vi "Test Cycle.vi"() -> ()   [LabVIEW 2018, in "TLMB.lvlib"]
uses:
  Projects/TLMB.lvlib
  Common/LabVIEW GEA2 Toolkit/GEA3/type defs/Source_Destination.ctl
  Common/LabVIEW GEA2 Toolkit/GEA3/type defs/ERD Read Data In.ctl
  Common/LabVIEW GEA2 Toolkit/GEA3/type defs/Data Type.ctl
  type defs/Drive Cycle Engine Request State.ctl
  type defs/Motor Control Without Stop Start.ctl
  Common/LabVIEW GEA2 Toolkit/GEA3/type defs/ERD Write Data In.ctl
  C:/Users/iallatyp/Desktop/New folder/GEA3/library/GEA2_Toolkit.lvlib
panel:
  in  "Spray Rinse Time (s)":dbl=120.0 caption="Delay Time (s)"
  in  "Intermediate Spin Time":dbl=120.0 caption="Delay Time (s)"
  in  "Agitate Time (s)":dbl=30.0 caption="Delay Time (s)"
  in  "Final Spin Time (s)":dbl=180.0 format="%#_13g"
  out "Error Out":errorcluster={"status"=TRUE, "code"=1172, "source"="Invoke Node Error calling method GeaCommunication.GeaBus.Read, (System.ArgumentNullException: Key cannot be null.\r\nParameter name: key) <append><b>System.ArgumentNullException</b> in LabVIEW_GEA2_Toolkit.lvlibp:GEA2 Send and Receive Message.vi->LabVIEW_GEA2_Toolkit.lvlibp:GEA2 Write ERD.vi->Drive Cycle Engine Request State ERD.vi->Test Cycle.vi"}
  in  "Target Gallons":dbl=4.0
  in  "Error In":errorcluster
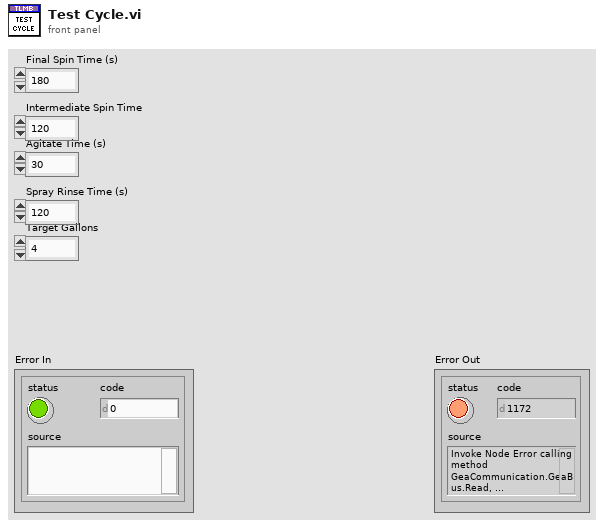
[diagram p1: front panel]
types:
  T1 = enum16{"EQ (==)", "NE (!=)", "GT (>)", "LT (<)", "GE (>=)", "LE (<=)", "GTLT(> <)", "GELE (>= <=)", "GELT (>= <)", "GTLE (> <=)", "LTGT (< >)", "LEGE (<= >=)", "LEGT (<= >)", "LTGE (< >=)", "No Comparison"}
  T2 = typedef "GEA2_Toolkit.lvlib/ERD Read Data In.ctl" = cluster{"ERD Number":u16, "Data Type":T3}
  T3 = typedef "GEA2_Toolkit.lvlib/Data Type.ctl" = enum16{"string", "boolean", "uint8_t", "uint16_t", "uint32_t", "uint64_t", "int8_t", "int16_t", "int32_t", "int64_t"}
  T4 = enum16{"ALL OFF", "Cold Valve", "Hot Valve", "Fabric Softener Valve", "Spray Rinse Valve", "Hot and Cold Valve"}
  T5 = typedef "GEA2_Toolkit.lvlib/ERD Write Data In.ctl" = cluster{"ERD Number":u16, "Data Type":T3, "Data":string}
  T6 = typedef "TLMB.lvlib/Drive Cycle Engine Request State.ctl" = enum16{"Start", "Stop", "Pause", "Resume", "Select"}
  T7 = typedef "TLMB.lvlib/Motor Control Without Stop Start.ctl" = cluster{"Speed (RPM)":i16, "Motor Profile Mode":u16, "Acceleration":i16, "Angle (Degrees)":i16, "Amplitude (%)\n-CCW +CW":i16}
  T8 = typedef "GEA2_Toolkit.lvlib/Source_Destination.ctl" = cluster{"Source":u8, "Destination":u8}
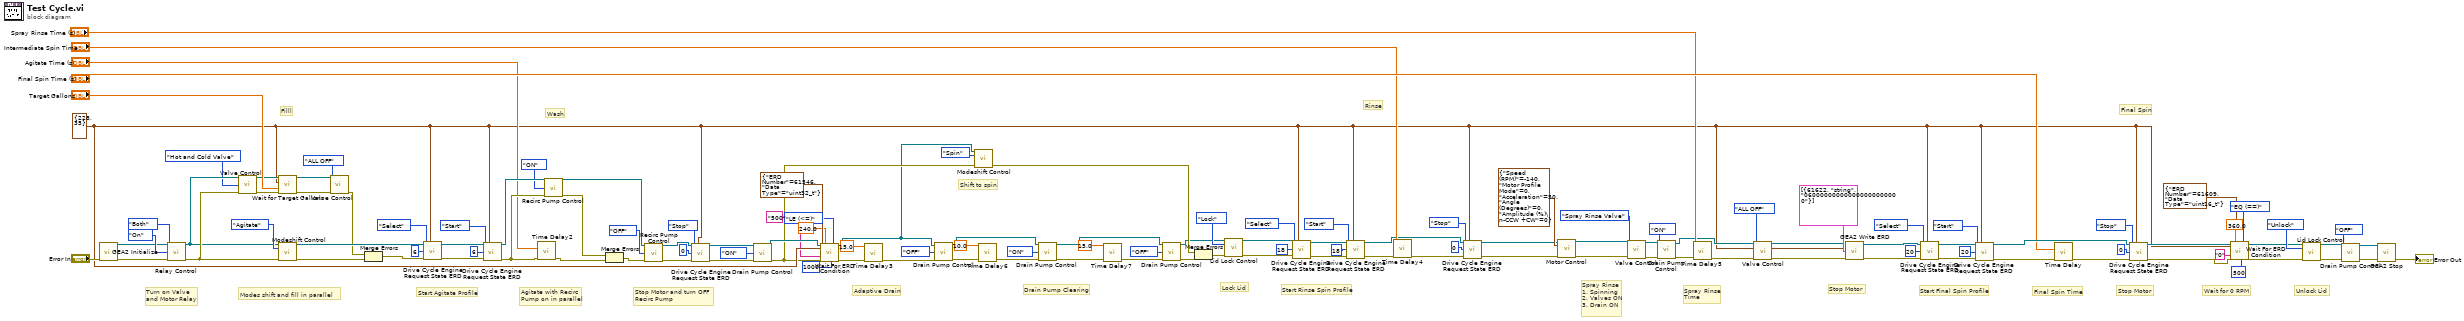
[diagram p0: block diagram]
diagram:
  w30 = T8 {"Source"=228, "Destination"=35} ("GEA Inputs")
  # "Drain Pump Clearing"
  # "Spray Rinse\n1. Spinning\n2. Valves ON\n3. Drain ON"
  # "Spray Rinse\nTime"
  # "Stop Motor"
  # "Start Rinse Spin Profile"
  # "Filll"
  # "Wash"
  # "Rinse"
  # "Final Spin"
  # "Final Spin Time"
  # "Unlock Lid"
  # "Stop Motor"
  # "Lock Lid"
  # "Shift to spin"
  # "Adaptive Drain"
  # "Stop Motor and turn OFF \nRecirc Pump"
  # "Agitate with Recirc\nPump on in parallel"
  # "Modes shift and fill in parallel"
  # "Wait for 0 RPM"
  # "Start Final Spin Profile"
  # "Start Agitate Profile"
  # "Turn on Valve \nand Motor Relay"
  n1 = call "GEA2 Initialize.vi"("error in"="Error In") -> ("GEA2 Reference Out"=w72:refnum<k24>, "error out"=w73:errorcluster)  [unwired: 12 in, 1 out]
  n2 = call "Relay Control.vi"("GEA2 Reference In"=w72, "Relay"=enum16{"Motor Enable", "Valve", "Both"}."Both", "State"=enum16{"On", "Off"}."On", "Error In"=w73) -> ("GEA2 Reference Out"=w121:refnum<k24>, "Error Out"=w122:errorcluster)  [unwired: 8 in, 2 out]
  n3 = call "Valve Control.vi"("GEA2 Reference In"=w121, "Fixed  Valve Control"=T4."Hot and Cold Valve", "Error In"=w122) -> ("GEA2 Reference Out"=w127:refnum<k24>, "Error Out"=w128:errorcluster)  [unwired: 11 in]
  n4 = call "Modeshift Control.vi"("GEA2 Reference In"=w121, "Shift To"=enum16{"Spin", "Agitate"}."Agitate", "Error In"=w122) -> ("GEA2 Reference Out"=w120:refnum<k24>, "Error Out"=w113:errorcluster)  [unwired: 9 in, 2 out]
  n5 = call "Wait for Target Gallons.vi"(".NET Refnum in"=w127, "GEA Inputs"=w30, "Target Gallons"="Target Gallons", "error in (no error)"=w128) -> ("GEA2 Reference Out"=w125:refnum<k24>, "error out"=w126:errorcluster)  [unwired: 10 in]
  n6 = call "Valve Control.vi"("GEA2 Reference In"=w125, "Fixed  Valve Control"=T4."ALL OFF", "Error In"=w126) -> ("Error Out"=w111:errorcluster)  [unwired: 11 in, 1 out]
  n7 = Merge Errors(w111, w113) -> (w112:errorcluster)
  n8 = call "Drive Cycle Engine Request State ERD.vi"("GEA2 Reference In"=w120, "GEA Inputs"=w30, "Cycle ID"=u8 6, "Drive Cycle Engine Request State"=Drive_Cycle_Engine_Request_State."Select", "Error In"=w112) -> ("GEA2 Reference Out"=w115:refnum<k24>, "Error Out"=w114:errorcluster)  [unwired: 9 in]
  n9 = call "Drive Cycle Engine Request State ERD.vi"("GEA2 Reference In"=w115, "GEA Inputs"=w30, "Cycle ID"=u8 6, "Drive Cycle Engine Request State"=Drive_Cycle_Engine_Request_State."Start", "Error In"=w114) -> ("GEA2 Reference Out"=w94:refnum<k24>, "Error Out"=w95:errorcluster)  [unwired: 9 in]
  n10 = call "Time Delay2"("error in (no error)"=w95, "Delay Time (s)"="Agitate Time (s)") -> ("error out"=w92:errorcluster)  [unwired: 9 in]
  n11 = call "Recirc Pump Control.vi"("GEA2 Reference In"=w94, "Drain Pump State"=enum16{"OFF", "ON"}."ON", "Error In"=w95) -> ("GEA2 Reference Out"=w88:refnum<k24>, "Error Out"=w91:errorcluster)  [unwired: 11 in]
  n12 = Merge Errors(w91, w92) -> (w90:errorcluster)
  n13 = call "Recirc Pump Control.vi"("GEA2 Reference In"=w88, "Drain Pump State"=enum16{"OFF", "ON"}."OFF", "Error In"=w90) -> ("GEA2 Reference Out"=w80:refnum<k24>, "Error Out"=w82:errorcluster)  [unwired: 11 in]
  n14 = call "Drive Cycle Engine Request State ERD.vi"("GEA2 Reference In"=w80, "GEA Inputs"=w30, "Cycle ID"=u8 0, "Drive Cycle Engine Request State"=Drive_Cycle_Engine_Request_State."Stop", "Error In"=w82) -> ("GEA2 Reference Out"=w79:refnum<k24>, "Error Out"=w81:errorcluster)  [unwired: 9 in]
  n15 = call "Drain Pump Control.vi"("GEA2 Reference In"=w79, "Drain Pump State"=enum16{"OFF", "ON"}."ON", "Error In"=w81) -> ("GEA2 Reference Out"=w31:refnum<k24>, "Error Out"=w11:errorcluster)  [unwired: 11 in]
  n16 = call "Wait For ERD Condition.vi"("GEA2 Reference In"=w31, "GEA Inputs"=w30, "ERD Read Data"=T2 {"ERD Number"=61546, "Data Type"=enum."uint32_t"}, "Expected Low"="500", "Error In"=w11, "Timeout (s)"=240.0, "Loop Rate (ms)"=u32 1000, "Comparison"=T1."LE (<=)") -> ("GEA2 Reference Out"=w1:refnum<k24>, "Error Out"=w23:errorcluster)  [unwired: 7 in, 3 out]
  n17 = call "Time Delay3"("error in (no error)"=w23, "Delay Time (s)"=15.0) -> ("error out"=w20:errorcluster)  [unwired: 9 in]
  n18 = call "Drain Pump Control.vi"("GEA2 Reference In"=w1, "Drain Pump State"=enum16{"OFF", "ON"}."OFF", "Error In"=w20) -> ("GEA2 Reference Out"=w4:refnum<k24>, "Error Out"=w19:errorcluster)  [unwired: 11 in]
  n19 = call "Modeshift Control.vi"("GEA2 Reference In"=w1, "Shift To"=enum16{"Spin", "Agitate"}."Spin", "Error In"=w11) -> ("Error Out"=w9:errorcluster)  [unwired: 9 in, 3 out]
  n20 = call "Time Delay6"("error in (no error)"=w19, "Delay Time (s)"=10.0) -> ("error out"=w17:errorcluster)  [unwired: 9 in]
  n21 = call "Drain Pump Control.vi"("GEA2 Reference In"=w4, "Drain Pump State"=enum16{"OFF", "ON"}."ON", "Error In"=w17) -> ("GEA2 Reference Out"=w3:refnum<k24>, "Error Out"=w13:errorcluster)  [unwired: 11 in]
  n22 = call "Time Delay7"("error in (no error)"=w13, "Delay Time (s)"=15.0) -> ("error out"=w16:errorcluster)  [unwired: 9 in]
  n23 = call "Drain Pump Control.vi"("GEA2 Reference In"=w3, "Drain Pump State"=enum16{"OFF", "ON"}."OFF", "Error In"=w16) -> ("GEA2 Reference Out"=w2:refnum<k24>, "Error Out"=w10:errorcluster)  [unwired: 11 in]
  n24 = Merge Errors(w9, w10) -> (w8:errorcluster)
  n25 = call "Lid Lock Control.vi"("GEA2 Reference In"=w2, "Action"=enum16{"Lock", "Unlock"}."Lock", "Error In"=w8) -> ("GEA2 Reference Out"=w59:refnum<k24>, "Error Out"=w63:errorcluster)  [unwired: 9 in, 2 out]
  n26 = call "Drive Cycle Engine Request State ERD.vi"("GEA2 Reference In"=w59, "GEA Inputs"=w30, "Cycle ID"=u8 18, "Drive Cycle Engine Request State"=Drive_Cycle_Engine_Request_State."Select", "Error In"=w63) -> ("GEA2 Reference Out"=w65:refnum<k24>, "Error Out"=w64:errorcluster)  [unwired: 9 in]
  n27 = call "Drive Cycle Engine Request State ERD.vi"("GEA2 Reference In"=w65, "GEA Inputs"=w30, "Cycle ID"=u8 18, "Drive Cycle Engine Request State"=Drive_Cycle_Engine_Request_State."Start", "Error In"=w64) -> ("GEA2 Reference Out"=w47:refnum<k24>, "Error Out"=w61:errorcluster)  [unwired: 9 in]
  n28 = call "Time Delay4"("error in (no error)"=w61, "Delay Time (s)"="Intermediate Spin Time") -> ("error out"=w50:errorcluster)  [unwired: 9 in]
  n29 = call "Drive Cycle Engine Request State ERD.vi"("GEA2 Reference In"=w47, "GEA Inputs"=w30, "Cycle ID"=u8 0, "Drive Cycle Engine Request State"=Drive_Cycle_Engine_Request_State."Stop", "Error In"=w50) -> ("GEA2 Reference Out"=w41:refnum<k24>, "Error Out"=w49:errorcluster)  [unwired: 9 in]
  n30 = call "Motor Control.vi"("GEA2 Reference In"=w41, "Motor Control"=T7 {"Speed (RPM)"=-140, "Motor Profile Mode"=0, "Acceleration"=50, "Angle (Degrees)"=0, "Amplitude (%)\n-CCW +CW"=0}, "Error In"=w49) -> ("GEA2 Reference Out"=w57:refnum<k24>, "Error Out"=w58:errorcluster)  [unwired: 11 in]
  n31 = call "Valve Control.vi"("GEA2 Reference In"=w57, "Fixed  Valve Control"=T4."Spray Rinse Valve", "Error In"=w58) -> ("GEA2 Reference Out"=w55:refnum<k24>, "Error Out"=w56:errorcluster)  [unwired: 11 in]
  n32 = call "Drain Pump Control.vi"("GEA2 Reference In"=w55, "Drain Pump State"=enum16{"OFF", "ON"}."ON", "Error In"=w56) -> ("GEA2 Reference Out"=w36:refnum<k24>, "Error Out"=w53:errorcluster)  [unwired: 11 in]
  n33 = call "Time Delay5"("error in (no error)"=w53, "Delay Time (s)"="Spray Rinse Time (s)") -> ("error out"=w39:errorcluster)  [unwired: 9 in]
  n34 = call "Valve Control.vi"("GEA2 Reference In"=w36, "Fixed  Valve Control"=T4."ALL OFF", "Error In"=w39) -> ("GEA2 Reference Out"=w37:refnum<k24>, "Error Out"=w38:errorcluster)  [unwired: 11 in]
  n35 = call "GEA2 Write ERD.vi"("GEA2 Reference In"=w37, "GEA Inputs"=w30, "Write ERD List"=T5[] [{"ERD Number"=61622, "Data Type"=enum."string", "Data"="060000000000000000000000"}], "Error In"=w38) -> ("GEA2 Reference Out"=w42:refnum<k24>, "Error Out"=w45:errorcluster)  [unwired: 9 in, 1 out]
  n36 = call "Drive Cycle Engine Request State ERD.vi"("GEA2 Reference In"=w42, "GEA Inputs"=w30, "Cycle ID"=u8 20, "Drive Cycle Engine Request State"=Drive_Cycle_Engine_Request_State."Select", "Error In"=w45) -> ("GEA2 Reference Out"=w109:refnum<k24>, "Error Out"=w110:errorcluster)  [unwired: 9 in]
  n37 = call "Drive Cycle Engine Request State ERD.vi"("GEA2 Reference In"=w109, "GEA Inputs"=w30, "Cycle ID"=u8 20, "Drive Cycle Engine Request State"=Drive_Cycle_Engine_Request_State."Start", "Error In"=w110) -> ("GEA2 Reference Out"=w96:refnum<k24>, "Error Out"=w85:errorcluster)  [unwired: 9 in]
  n38 = call "Time Delay"("error in (no error)"=w85, "Delay Time (s)"="Final Spin Time (s)") -> ("error out"=w71:errorcluster)  [unwired: 9 in]
  n39 = call "Drive Cycle Engine Request State ERD.vi"("GEA2 Reference In"=w96, "GEA Inputs"=w30, "Cycle ID"=u8 0, "Drive Cycle Engine Request State"=Drive_Cycle_Engine_Request_State."Stop", "Error In"=w71) -> ("GEA2 Reference Out"=w76:refnum<k24>, "Error Out"=w75:errorcluster)  [unwired: 9 in]
  n40 = call "Wait For ERD Condition.vi"("GEA2 Reference In"=w76, "GEA Inputs"=w30, "ERD Read Data"=T2 {"ERD Number"=61609, "Data Type"=enum."uint16_t"}, "Expected Low"="0", "Error In"=w75, "Timeout (s)"=360.0, "Loop Rate (ms)"=u32 500, "Comparison"=T1."EQ (==)") -> ("GEA2 Reference Out"=w97:refnum<k24>, "Error Out"=w98:errorcluster)  [unwired: 7 in, 3 out]
  n41 = call "Lid Lock Control.vi"("GEA2 Reference In"=w97, "Action"=enum16{"Lock", "Unlock"}."Unlock", "Error In"=w98) -> ("GEA2 Reference Out"=w43:refnum<k24>, "Error Out"=w44:errorcluster)  [unwired: 9 in, 2 out]
  n42 = call "Drain Pump Control.vi"("GEA2 Reference In"=w43, "Drain Pump State"=enum16{"OFF", "ON"}."OFF", "Error In"=w44) -> ("GEA2 Reference Out"=w5:refnum<k24>, "Error Out"=w7:errorcluster)  [unwired: 11 in]
  n43 = call "GEA2 Stop.vi"("GEA2 Reference In"=w5, "Error In"=w7) -> ("Error Out"=→"Error Out":errorcluster)  [unwired: 13 in]
